vi "Add_Inlet_Temp_at_Z.vi"() -> (5 "Plug in titles":string[](array[string]), 7 "Plug in values":string[](array[string]))   [LabVIEW 2015]
uses:
  Globals/Meas_global.vi
panel:
  out "Z":dbl
  # "Please enter any run information in the box below"
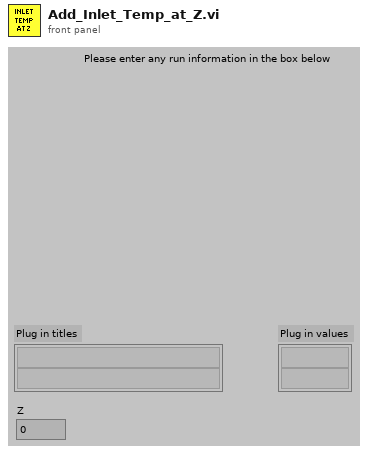
[diagram p1: front panel]
types:
  T1 = typedef "Analysis_info_cluster.ctl" = cluster{"Colour":u32, "Inst type":T2, "Inst name":string, "Symbol":string, "Code name":string, "Extra Info":string, "Inst Array":T3, "Extra Titles":string[], "Extra Values":string[], "U":dbl, "u^2":dbl, "u^3":dbl, "u^4":dbl, "Skew_u":dbl, "Kurt_u":dbl, "Sd Error in Mean":dbl, "% u'/U":dbl, "X":dbl, "Y":dbl, "Z":dbl, "Timescale integral to 25%":dbl, "Sd Error in Variance":dbl, "Calib File":path, "Calib Constants":dbl[], "Output Position":bool, "Full Stats":bool, "Av Sampling Rate":dbl, "Av No of Samples":dbl, "Total Meas Time (s)":dbl, "ADAM Ch Name":string}
  T2 = typedef "Inst_type.ctl" = enum16{"Propeller anemometer", "Raw voltage", "Pressure Transducer", "Pitot-static tube", "Preston tube", "Hot wire", "Cross wire 1", "Cross wire 2", "Generic Linear", "Generic Polynomial", "Generic BackPoly", "Fast FID", "Thermocouple", "Cold wire", "Pulsed Wire", "LDA Vel", "LDA Tran time", "LDA Arr time", "Microphone"}
  T3 = typedef "Instrument_Array.ctl" = enum16{"PWA", "LDA", "Analogue"}
  T4 = typedef "Post_Process.ctl" = enum16{"Take New Data", "Post Process Raw Data File"}
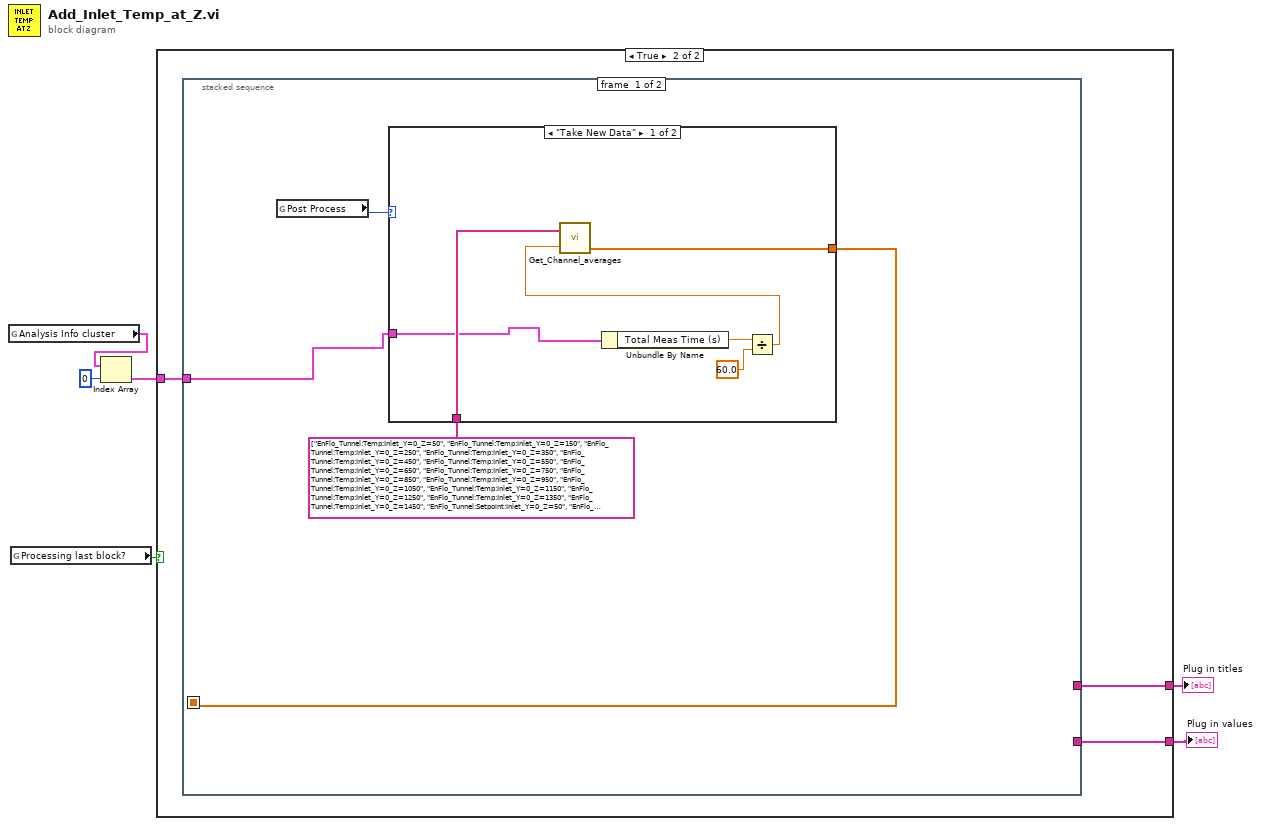
[diagram p0: block diagram]
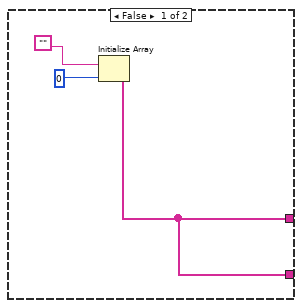
[diagram p2: hidden frame]
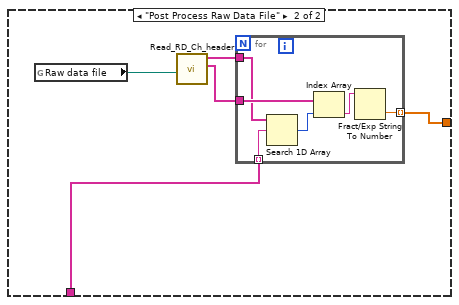
[diagram p3: hidden frame]
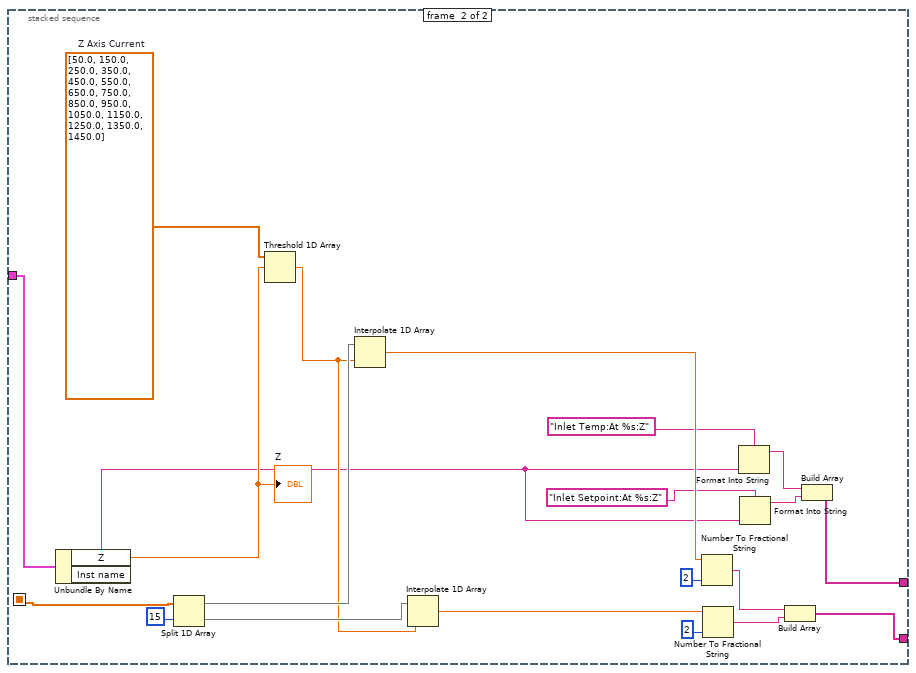
[diagram p4: hidden frame]
diagram:
  n1 = global read "Meas_global.vi" "Analysis Info cluster"() -> (w2:T1[])
  n2 = global read "Meas_global.vi" "Processing last block?"() -> (w6:bool)
  n3 = Index Array(array=w2, index=0) -> (element=w1:T1)
  n4 = case shown="True" w6 {
    tunnel: [w7 w11] -> w5
    tunnel: [w7 w12] -> w4
    tunnel: w1 -> [_ w10]
    frame False {
      n5 = Initialize Array("", 0) -> (w7:string[])
    }
    frame True {
      n6 = stacked-sequence {
        seq-local: [w14 _] -> [_ w46]
        tunnel: [_ w51] -> w12
        tunnel: [_ w50] -> w11
        tunnel: w10 -> [w13 w34]
        frame #0 {
          n7 = global read "Meas_global.vi" "Post Process"() -> (w16:T4)
          n8 = case shown="\"Take New Data\"" w16 {
            tunnel: string[] ["EnFlo_Tunnel:Temp:Inlet_Y=0_Z=50", "EnFlo_Tunnel:Temp:Inlet_Y=0_Z=150", "EnFlo_Tunnel:Temp:Inlet_Y=0_Z=250", "EnFlo_Tunnel:Temp:Inlet_Y=0_Z=350", "EnFlo_Tunnel:Temp:Inlet_Y=0_Z=450", "EnFlo_Tunnel:Temp:Inlet_Y=0_Z=550", "EnFlo_Tunnel:Temp:Inlet_Y=0_Z=650", "EnFlo_Tunnel:Temp:Inlet_Y=0_Z=750", "EnFlo_Tunnel:Temp:Inlet_Y=0_Z=850", "EnFlo_Tunnel:Temp:Inlet_Y=0_Z=950", "EnFlo_Tunnel:Temp:Inlet_Y=0_Z=1050", "EnFlo_Tunnel:Temp:Inlet_Y=0_Z=1150", "EnFlo_Tunnel:Temp:Inlet_Y=0_Z=1250", "EnFlo_Tunnel:Temp:Inlet_Y=0_Z=1350", "EnFlo_Tunnel:Temp:Inlet_Y=0_Z=1450", "EnFlo_Tunnel:Setpoint:Inlet_Y=0_Z=50", "EnFlo_Tunnel:Setpoint:Inlet_Y=0_Z=150", "EnFlo_Tunnel:Setpoint:Inlet_Y=0_Z=250", "EnFlo_Tunnel:Setpoint:Inlet_Y=0_Z=350", "EnFlo_Tunnel:Setpoint:Inlet_Y=0_Z=450", "EnFlo_Tunnel:Setpoint:Inlet_Y=0_Z=550", "EnFlo_Tunnel:Setpoint:Inlet_Y=0_Z=650", "EnFlo_Tunnel:Setpoint:Inlet_Y=0_Z=750", "EnFlo_Tunnel:Setpoint:Inlet_Y=0_Z=850", "EnFlo_Tunnel:Setpoint:Inlet_Y=0_Z=950", "EnFlo_Tunnel:Setpoint:Inlet_Y=0_Z=1050", "EnFlo_Tunnel:Setpoint:Inlet_Y=0_Z=1150", "EnFlo_Tunnel:Setpoint:Inlet_Y=0_Z=1250", "EnFlo_Tunnel:Setpoint:Inlet_Y=0_Z=1350", "EnFlo_Tunnel:Setpoint:Inlet_Y=0_Z=1450"] ("Sub set") -> [w22 w24]
            tunnel: [w21 w23] -> w14
            tunnel: w13 -> [w17 _]
            frame "Take New Data" {
              n9 = Unbundle By Name(w17) -> ("Total Meas Time (s)"=w20:dbl)
              n10 = Divide(x=w20, y=60.0) -> (x/y=w18:dbl)
              n11 = call "Get_Channel_averages.vi"("Desired Ch Names"=w22, "Averaging time (mins)"=w18) -> ("number"=w21:dbl[])  [unwired: 1 in, 2 out]
            }
            frame "Post Process Raw Data File" {
              n12 = global read "Meas_global.vi" "Raw data file"() -> (w27:path)
              n13 = call "Read_RD_Ch_header.vi"("Raw data file"=w27) -> ("Ch Name Out"=w25:string[], "Ch Values"=w26:string[])  [unwired: 2 out]
              n14 = for {
                tunnel: w26 -> [w33]
                tunnel: w25 -> [w32]
                tunnel: w24 -> [w31] mode=indexing
                tunnel: [w28] -> w23 mode=indexing
                n15 = Search 1D Array(1D array=w32, element=w31) -> (index of element=w30:i32)  [unwired: 1 in]
                n16 = Index Array(array=w33, index=w30) -> (element=w29:string)
                n17 = Fract/Exp String To Number(string=w29) -> (number=w28:dbl)  [unwired: 3 in, 1 out]
              }
            }
          }
        }
        frame #1 {
          w54 = dbl[] [50.0, 150.0, 250.0, 350.0, 450.0, 550.0, 650.0, 750.0, 850.0, 950.0, 1050.0, 1150.0, 1250.0, 1350.0, 1450.0]  # Z Axis Current
          n18 = Unbundle By Name(w34) -> ("Z"=w53:dbl, "Inst name"=w39:string)
          "Z" <- w53
          n19 = Split 1D Array(array=w46, index=15) -> (first subarray=w44:dbl[], second subarray=w43:dbl[])
          n20 = Threshold 1D Array(2:w53, 3:w54) -> (0:w42:dbl)  [unwired: 1 in]
          n21 = Interpolate 1D Array(1:w42, 2:w44) -> (0:w52:dbl)
          n22 = Interpolate 1D Array(1:w42, 2:w43) -> (0:w35:dbl)
          n23 = Number To Fractional String(number=w52, precision (6)=i16 2) -> (F-format string=w41:string)  [unwired: 2 in]
          n24 = Number To Fractional String(number=w35, precision (6)=i16 2) -> (F-format string=w36:string)  [unwired: 2 in]
          n25 = Format Into String(format string="Inlet Temp:At %s:Z", w39) -> (resulting string=w48:string)  [unwired: 2 in, 1 out]
          n26 = Format Into String(format string="Inlet Setpoint:At %s:Z", w39) -> (resulting string=w38:string)  [unwired: 2 in, 1 out]
          n27 = Build Array(w41, w36) -> (w51:string[])
          n28 = Build Array(w48, w38) -> (w50:string[])
        }
      }
    }
  }
  "Plug in titles" <- w5
  "Plug in values" <- w4
